vi "OpenXL_App.vi"(8 "error in (no error)":errorcluster) -> (0 "error out":errorcluster, 3 "Refnum Cluster":T1)   [LabVIEW 2015]
doc: "This VI opens up an Excel Application object. Multiple workbooks and worksheets can be opened within the same Application session. Always pair this VI with a Close XL Application VI."
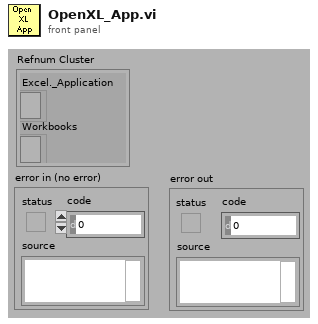
[diagram p1: front panel]
types:
  T1 = cluster{"Excel._Application":refnum<k7>, "Workbooks":refnum<k7>}
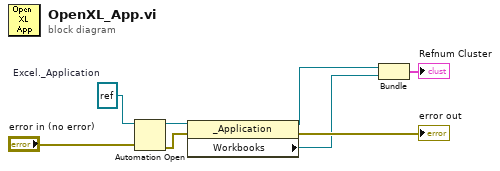
[diagram p0: block diagram]
diagram:
  w6 = refnum<k7> refnum  # Excel._Application
  n1 = Automation Open(error in (no error)="error in (no error)", Automation Refnum=w6) -> (Automation Refnum=w2:refnum<k7>, error out=w7:errorcluster)  [unwired: 2 in]
  n2 = property class="_Application"(reference=w2, error in=w7) -> (reference out=w5:refnum<k7>, error out=→"error out":errorcluster, "Workbooks"=w4:refnum<k7>)
  n3 = Bundle("Excel._Application"=w5, "Workbooks"=w4) -> (→"Refnum Cluster":T1)  [unwired: 1 in]
